vi "Limight LED OFF.vi"(11 "LED OFF":bool) -> ()   [LabVIEW 2019]
uses:
  <vilib>/Rock Robotics/Network Tables/NT Write Number.vi
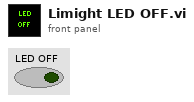
[diagram p1: front panel]
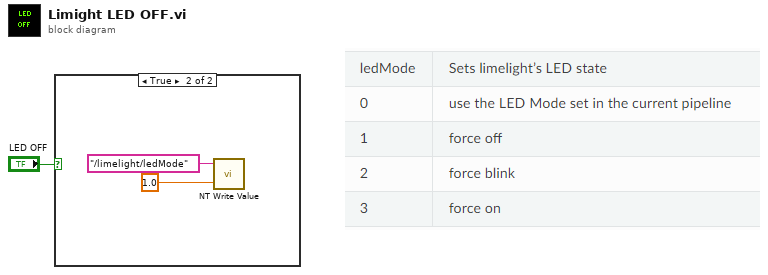
[diagram p0: block diagram]
diagram:
  n1 = case shown="True" "LED OFF" {
    frame False {
    }
    frame True {
      n2 = call-poly <vilib>:"NT Write Value.vi"("Numeric"=1.0, "Name"="/limelight/ledMode") -> ()  [unwired: 9 in, 1 out]
    }
  }
